vi "open configuration.vi"(4 "error in":errorcluster, 6 "file path":path, 7 "Sensor Array":T1) -> (0 "error out":errorcluster, 3 "Sensor Array out":T1)   [LabVIEW 2012]
uses:
  DAQ configuration/Sensor array.ctl
  DAQ configuration/channel identifier.ctl
  file action.ctl
  calibration/global scale array.vi
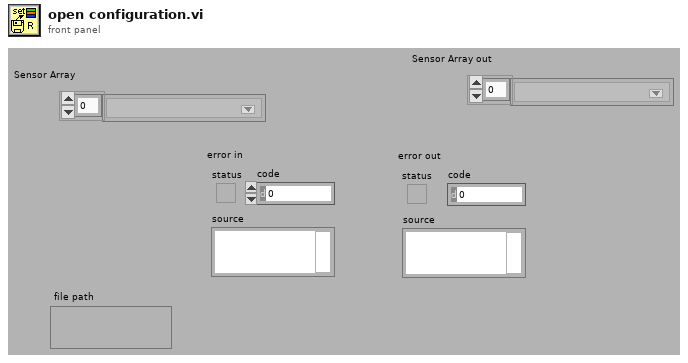
[diagram p1: front panel]
types:
  T1 = typedef "Sensor array.ctl" = T2[]
  T2 = typedef "channel identifier.ctl" = u16
  T3 = typedef "file action.ctl" = enum16{"Save", "Open"}
  T4 = typedef "calib array.ctl" = T5[]
  T5 = typedef "conversion.ctl" = cluster{"conversion matrix":sgl[][], "units":string, "name":string, "scale type":T6, "offset (volts)":dbl, "second channel":i8, "correspondence table":T7, "offset (physical units)":dbl, "pH scale":T8, "D.O.":T9}
  T6 = typedef "scale type.ctl" = enum16{"Volts", "Polynomial", "Correspondence Table", "pH", "Dissolved Oxygen", "Quadratic"}
  T7 = typedef "correspondence table.ctl" = cluster{"physical units":dbl, "volts":dbl}[]
  T8 = typedef "pH scale.ctl" = cluster{"Buffers":cluster{"Buffer":dbl, "Calibrated":bool, "V/T":dbl}[], "Temperature":dbl}
  T9 = typedef "DO scale.ctl" = cluster{"Temperature":dbl, "K":dbl, "barometric pressure":dbl}
  T10 = cluster{"Sensor Array":T1, "Calibration matrix":T4}
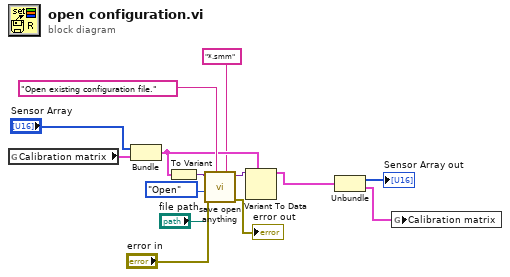
[diagram p0: block diagram]
diagram:
  n1 = global read "global scale array.vi" "Calibration matrix"() -> (w9:T4)
  n2 = Bundle("Sensor Array"="Sensor Array", "Calibration matrix"=w9) -> (w8:T10)  [unwired: 1 in]
  n3 = To Variant(anything=w8) -> (Variant=w13:variant)
  n4 = call "save open anything.vi"("Variant"=w13, "file path"="file path", "Action"=file_action."Open", "error in (not an error)"="error in", "prompt"="Open existing configuration file.", "pattern"="*.smm") -> ("Variant out"=w14:variant, "error out"=→"error out":errorcluster)  [unwired: 1 in, 2 out]
  n5 = Variant To Data(type=w8, Variant=w14) -> (data=w7:T10)  [unwired: 1 in, 1 out]
  n6 = Unbundle(w7) -> ("Sensor Array"=→"Sensor Array out":T1, "Calibration matrix"=w6:T4)
  n7 = global write "global scale array.vi" "Calibration matrix"(w6) -> ()
